vi "Update Worktable Positions.vi"(8 "error in":errorcluster, 11 "Potting Procedure in":refnum<class "Potting Procedure.lvclass">) -> (0 "error out":errorcluster, 3 "Potting Procedure out":refnum<class "Potting Procedure.lvclass">)   [LabVIEW 2017, in "Potting Procedure.lvclass"]
uses:
  Potting Procedure.lvclass
  Shared Components/WorkTable Class/WorkTable Class.lvclass
  Shared Components/Config Manager Class/Config Manager Class.lvclass
  Shared Components/Gantry Class/Gantry Class.lvclass
  Shared Components/Config Manager Class/Type Definitions/Fiducial Type.ctl
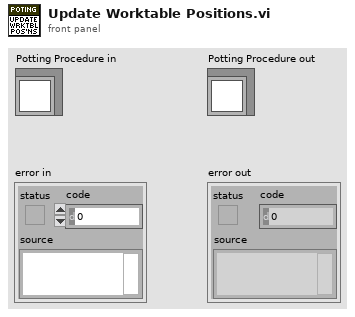
[diagram p1: front panel]
types:
  T1 = typedef "Fiducial Type.ctl" = enum16{"HDI", "BBM"}
  T2 = enum16{"Empty", "Bare HDI", "Unglued", "Stamped", "PartOnTop", "Weighted", "Unpotted", "Potted"}
  T3 = typedef "Inspect Fiducials.ctl" = cluster{"Has Been Run?":bool, "Module-Chuck Fiducials":cluster{"Fiducials-HDI":T4[], "Fiducials-BBM":T4[], "Chuck":i32, "Slot":i32}[]}
  T4 = typedef "Fiducial Image.ctl" = cluster{"Fiducial Image":T5, "Selected Fiducial":T7, "fiducial name":string}
  T5 = typedef "Physical Image.ctl" = cluster{"Image Position":refnum<class "Vec3d Class.lvclass">, "Image Reference":T6, "Field of View":cluster{"x(mm)":dbl, "y(mm)":dbl}}
  T6 = typedef "IMAQ Image.ctl" = refnum<image>
  T7 = typedef "Fiducial with Source.ctl" = cluster{"Fiducial Image Coordinate":refnum<class "Vec3d Class.lvclass">, "Fiducial Source":enum16{"Pattern Recognition", "User", "Error", "Default"}}
  T8 = cluster{"Fiducials-HDI":T4[], "Fiducials-BBM":T4[], "Chuck":i32, "Slot":i32}[]
  T9 = cluster{"Feature Coordinates":refnum<class "Vec3d Class.lvclass">, "Feature Name":string}[]
  T10 = typedef "Position_Orientation.ctl" = cluster{"Center":refnum<class "Vec3d Class.lvclass">, "Orientation":refnum<class "Orient3d Class.lvclass">}
  T11 = typedef "Worktable_Module Slot.ctl" = cluster{"Slot State":enum16{"Empty", "Bare HDI", "Unglued", "Stamped", "PartOnTop", "Weighted", "Unpotted", "Potted"}, "BBM Type":enum16{"None", "BBM", "GlassSlide"}, "HDI Type":enum16{"None", "HDI", "Polyimide"}, "Vacuum Channel":u8, "Location/Orientation BBM":T10, "Location/Orientation HDI":T10, "S/N":string}
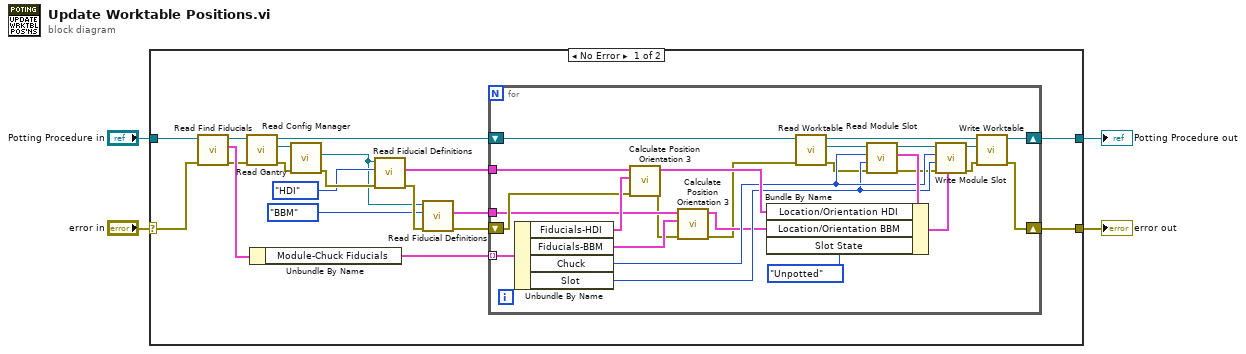
[diagram p0: block diagram]
diagram:
  n1 = case shown="No Error" "error in" {
    selector: "error in" -> [w14 w50]
    tunnel: [w8 w50] -> w3
    tunnel: [w15 w49] -> w1
    tunnel: "Potting Procedure in" -> [w23 w49]
    frame No Error {
      n2 = call-dynamic "Read Find Fiducials.vi"("error in (no error)"=w14, "Potting Procedure in"=w23) -> ("error out"=w13:errorcluster, "Find Fiducials"=w22:T3, "Potting Procedure out"=w12:refnum<class "Potting Procedure.lvclass">)  [unwired: 7 in]
      n3 = call-dynamic "Read Gantry.vi"("error in (no error)"=w13, "Potting Procedure in"=w12) -> ("error out"=w11:errorcluster, "Gantry"=w20:refnum<class "Gantry Class.lvclass">, "Potting Procedure out"=w16:refnum<class "Potting Procedure.lvclass">)  [unwired: 7 in]
      n4 = Unbundle By Name(w22) -> ("Module-Chuck Fiducials"=w21:T8)
      n5 = call-dynamic "Read Config Manager.vi"("error in"=w11, "Gantry in"=w20) -> ("error out"=w10:errorcluster, "Config Manager"=w5:refnum<class "Config Manager Class.lvclass">)  [unwired: 7 in, 1 out]
      n6 = call "Read Fiducial Definitions.vi"("error in"=w10, "Fiducial Type"=Fiducial_Type."HDI", "Config Manager in"=w5) -> ("error out"=w19:errorcluster, "Feature Definitions"=w17:T9)  [unwired: 6 in, 1 out]
      n7 = call "Read Fiducial Definitions.vi"("error in"=w19, "Fiducial Type"=Fiducial_Type."BBM", "Config Manager in"=w5) -> ("error out"=w9:errorcluster, "Feature Definitions"=w18:T9)  [unwired: 6 in, 1 out]
      n8 = for {
        tunnel: w21 -> [w48] mode=indexing
        tunnel: w18 -> [w33]
        tunnel: w17 -> [w46]
        shift-right: [w41] -> w15
        shift-left: w16 -> [w44]
        shift-right: [w25] -> w8
        shift-left: w9 -> [w45]
        n9 = Unbundle By Name(w48) -> ("Fiducials-HDI"=w47:T4[], "Fiducials-BBM"=w32:T4[], "Chuck"=w35:i32, "Slot"=w34:i32)
        n10 = call "Calculate Position Orientation 3.vi"("error in"=w45, "Fiducials"=w47, "Feature Definitions"=w46) -> ("error out"=w31:errorcluster, "PositionOrientation"=w36:T10)  [unwired: 7 in]
        n11 = call "Calculate Position Orientation 3.vi"("error in"=w31, "Fiducials"=w32, "Feature Definitions"=w33) -> ("error out"=w29:errorcluster, "PositionOrientation"=w30:T10)  [unwired: 7 in]
        n12 = call-dynamic "Read Worktable.vi"("error in"=w29, "Potting Procedure in"=w44) -> ("error out"=w28:errorcluster, "WorkTable out"=w39:refnum<class "WorkTable Class.lvclass">, "Potting Procedure out"=w43:refnum<class "Potting Procedure.lvclass">)  [unwired: 7 in]
        n13 = call-dynamic "Read Module Slot.vi"("error in"=w28, "slot"=w34, "chuck"=w35, "WorkTable in"=w39) -> ("error out"=w27:errorcluster, "Module Slot"=w37:T11, "WorkTable out"=w38:refnum<class "WorkTable Class.lvclass">)  [unwired: 5 in]
        n14 = Bundle By Name(cluster=w37, "Location/Orientation HDI"=w36, "Location/Orientation BBM"=w30, "Slot State"=T2."Unpotted") -> (w40:T11)
        n15 = call-dynamic "Write Module Slot.vi"("Module Slot"=w40, "error in"=w27, "slot"=w34, "chuck"=w35, "WorkTable in"=w38) -> ("error out"=w26:errorcluster, "WorkTable out"=w42:refnum<class "WorkTable Class.lvclass">)  [unwired: 5 in]
        n16 = call-dynamic "Write Worktable.vi"("error in"=w26, "WorkTable in"=w42, "Potting Procedure in"=w43) -> ("error out"=w25:errorcluster, "Potting Procedure out"=w41:refnum<class "Potting Procedure.lvclass">)  [unwired: 7 in]
      }
    }
    frame Error {
    }
  }
  "error out" <- w3
  "Potting Procedure out" <- w1
